vi "VI AK.vi"() -> (0 "error out":errorcluster)   [LabVIEW 2020, in "AK-Schnittstelle.lvlib"]
uses:
  AK-Schnittstelle.lvlib
  Aktionen AK.ctl
  Aktionen Gespeicherte Werte.ctl
  Allgemein/Zykluszeiterfassung Aktionen.ctl
  SysLog/SysLog Interface.ctl
  AK Seriell/AK Seriell.lvlib
  AK TCP/AK TCP.lvlib
  Allgemein/allgemeine Sub-VIs.lvlib
  SysLog/SysLog.lvlib
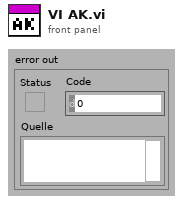
[diagram p1: front panel]
types:
  T1 = typedef "AK-Schnittstelle.lvlib/Aktionen AK.ctl" = enum16{"lesen", "initialisieren", "beenden", "AK Komm"}
  T2 = typedef "allgemeine Sub-VIs.lvlib/Zykluszeiterfassung Aktionen.ctl" = enum16{"lesen", "init", "Messdaten1", "ToolWeb", "AK FT-IR", "AK Extern", "AK Amium"}
  T3 = typedef "AK-Schnittstelle.lvlib/Aktionen Gespeicherte Werte.ctl" = enum16{"lesen", "laden", "speichern", "Seriell", "TCP", "Diverse", "AKTIV", "AK-Namen"}
  T4 = typedef "SysLog.lvlib/SysLog Interface.ctl" = cluster{"FehlermeldungsCode":i32, "ErfolgsmeldungsCode":i32, "ParameterListenString":string, "Anzeige":bool, "SysLogIcon":enum16{"OK", "Warnung", "Fehler"}, "intern":bool}
  T5 = typedef "AK-Schnittstelle.lvlib/AK TCP.lvlib/TCP Parameter.ctl" = cluster{"Port":u16, "Timeout":u16}
  T6 = typedef "AK-Schnittstelle.lvlib/AK Seriell.lvlib/Serielle Parameter.ctl" = cluster{"VISA resource name":refnum<visa-resource-name>, "baud rate":u32, "data bits":u16, "parity":u16, "stop bits":u16, "flow control":u16}
  T7 = cluster{"VISA resource name":bool, "baud rate":bool, "data bits":bool, "parity":bool, "stop bits":bool, "flow control":bool}
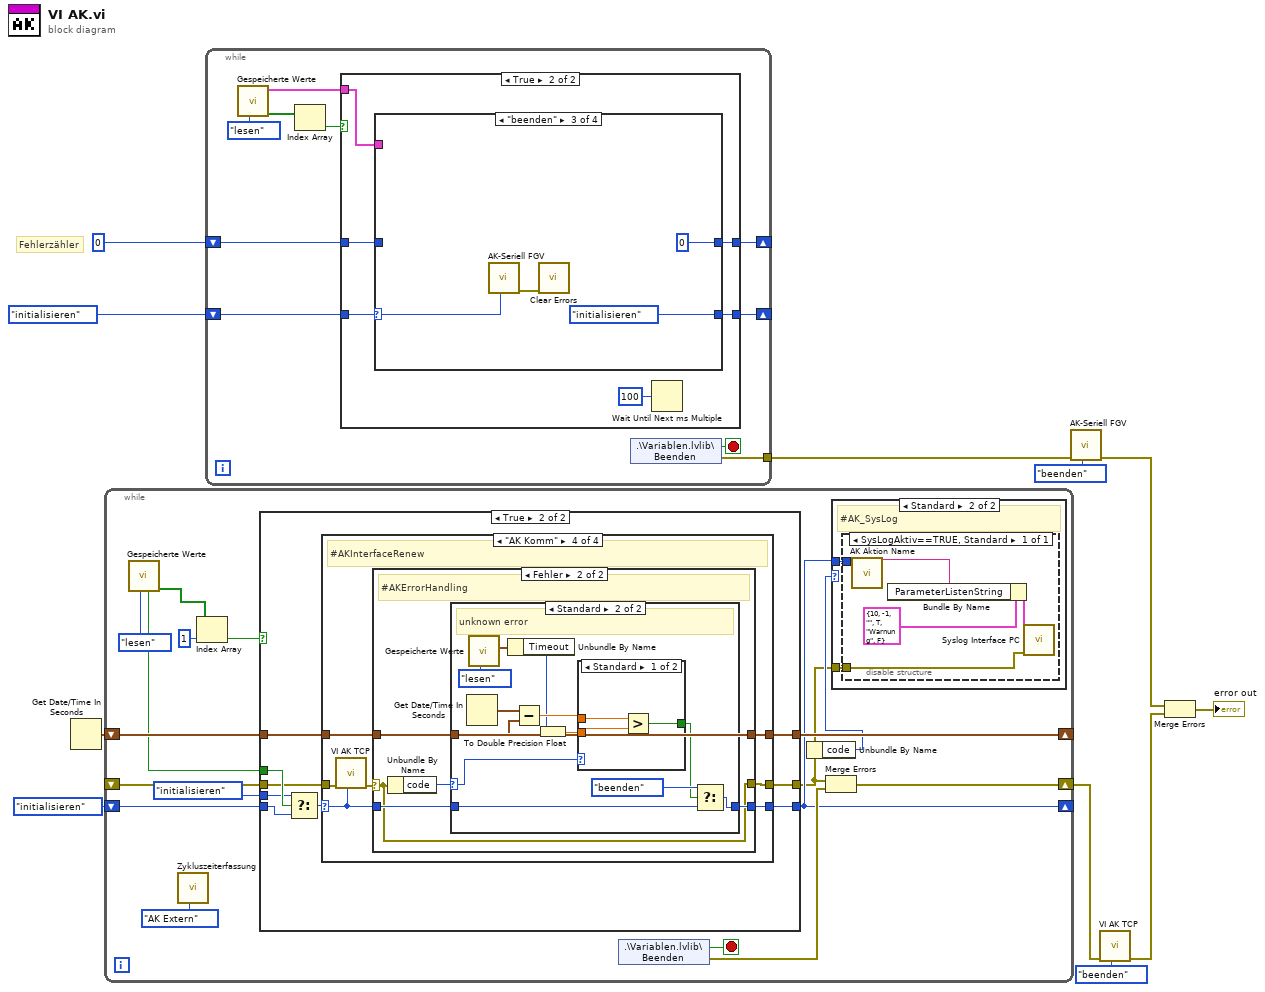
[diagram p0: block diagram]
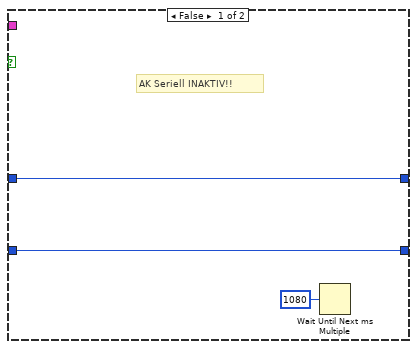
[diagram p2: hidden frame]
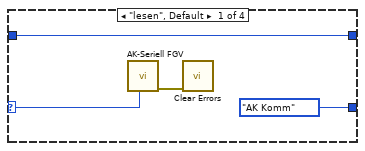
[diagram p3: hidden frame]
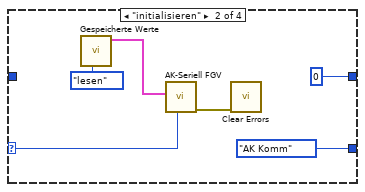
[diagram p4: hidden frame]
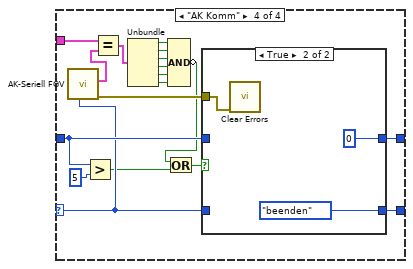
[diagram p5: hidden frame]
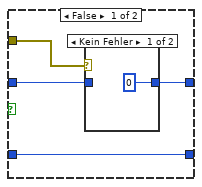
[diagram p6: hidden frame]
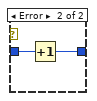
[diagram p7: hidden frame]
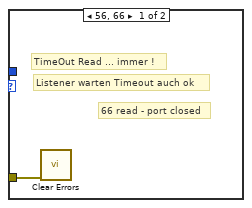
[diagram p8: hidden frame]
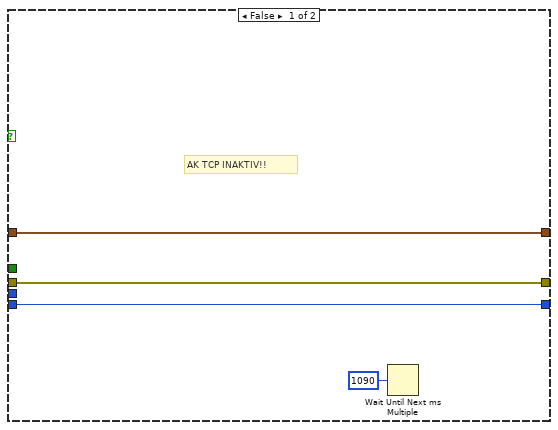
[diagram p9: hidden frame]
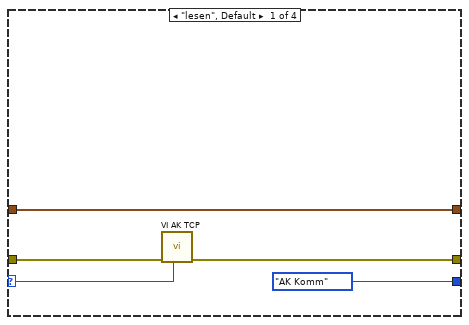
[diagram p10: hidden frame]
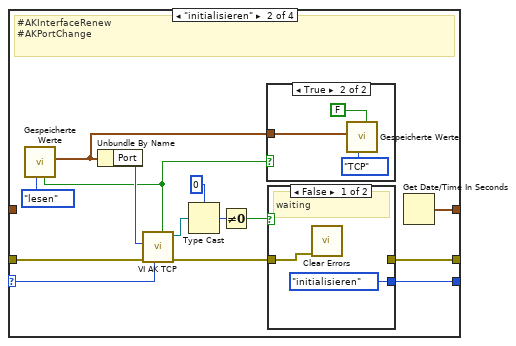
[diagram p11: hidden frame]
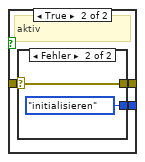
[diagram p12: hidden frame]
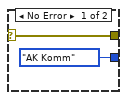
[diagram p13: hidden frame]
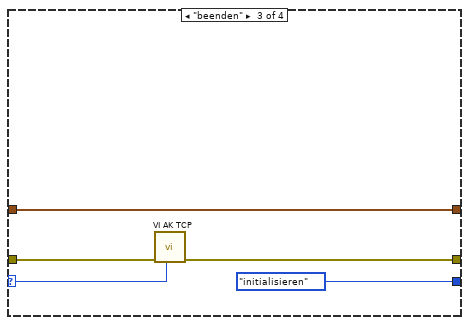
[diagram p15: hidden frame]
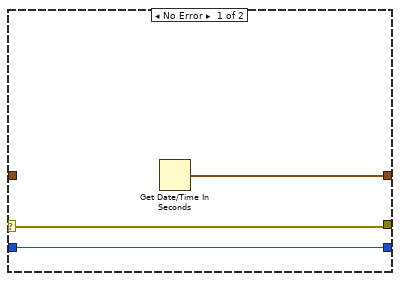
[diagram p16: hidden frame]
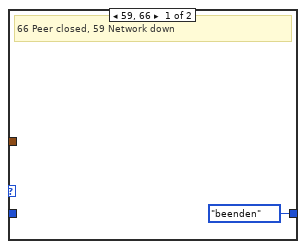
[diagram p17: hidden frame]
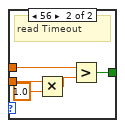
[diagram p18: hidden frame]
diagram:
  # "Fehlerzähler"
  n1 = Get Date/Time In Seconds() -> (seconds since 1Jan1904=w2:timestamp)
  n2 = while {
    shift-right: [w14] -> _
    shift-left: Aktionen_AK."initialisieren" ("Aktionen") -> [w28]
    shift-right: [w27] -> _
    shift-left: w2 -> [w26]
    shift-right: [w16] -> w1
    shift-left: _ -> [w15]
    stop <- w21 stop-if-true
    n3 = call "Gespeicherte Werte.vi"("Aktionen"=Aktionen_Gespeicherte_Werte."lesen") -> ("AKTIV?"=w24:bool[], "Port changed out"=w19:bool)  [unwired: 6 in, 3 out]
    n4 = call "Zykluszeiterfassung.vi"("Aktionen"=Zykluszeiterfassung_Aktionen."AK Extern") -> ()  [unwired: 10 in, 1 out]
    n5 = Index Array(array=w24, index=1 ("Index")) -> (element=w22:bool)
    n6 = case shown="True" w22 {
      tunnel: w28 -> [w39 w45]
      tunnel: [w39 w49] -> w14
      tunnel: [w40 w48] -> w27
      tunnel: w26 -> [w40 w47]
      tunnel: w19 -> [_ w46]
      tunnel: Aktionen_AK."initialisieren" ("Aktionen") -> [_ w44]
      tunnel: [w37 w42] -> w12
      tunnel: w15 -> [w37 w41]
      frame False {
        # "AK TCP INAKTIV!!"
        n7 = Wait Until Next ms Multiple(millisecond multiple=u32 1090 ("Vielfache von ms")) -> ()  [unwired: 1 out]
      }
      frame True {
        n8 = Select(t=w44, s=w46, f=w45) -> (s? t:f=w43:T1)
        n9 = case shown="\"AK Komm\"" w43 {
          selector: w43 -> [w52 w67 w84 w89]
          tunnel: [Aktionen_AK."AK Komm" ("Aktionen") w65 Aktionen_AK."initialisieren" ("Aktionen") w88] -> w49
          tunnel: [w53 w63 w83 w92] -> w48
          tunnel: w47 -> [w53 _ w83 w91]
          tunnel: [w50 w58 w81 w86] -> w42
          tunnel: w41 -> [w51 w57 w82 w87]
          frame "lesen", Default {
            n10 = call "VI AK TCP.vi"("Aktionen"=w52, "error in"=w51) -> ("error out"=w50:errorcluster)  [unwired: 8 in, 1 out]
          }
          frame "initialisieren" {
            # "#AKInterfaceRenew\n#AKPortChange"
            n11 = call "Gespeicherte Werte.vi"("Aktionen"=Aktionen_Gespeicherte_Werte."lesen") -> ("TCP Parameter"=w59:T5, "Port changed out"=w55:bool)  [unwired: 6 in, 3 out]
            n12 = Unbundle By Name(w59) -> ("Port"=w64:u16)
            n13 = call "VI AK TCP.vi"("Port changed in"=w55, "Aktionen"=w67, "error in"=w57, "Port"=w64) -> ("error out"=w66:errorcluster, "connection ID"=w56:refnum<k5>)  [unwired: 6 in]
            n14 = Type Cast(type=u32 0, x=w56) -> (*(type *) &x=w61:u32)
            n15 = Not Equal To 0?(x=w61) -> (x != 0?=w60:bool)
            n16 = case shown="True" w55 {
              tunnel: w59 -> [_ w78]
              frame False {
              }
              frame True {
                n17 = call "Gespeicherte Werte.vi"("Port changed in"=FALSE, "Aktionen"=Aktionen_Gespeicherte_Werte."TCP", "TCP Parameter"=w78) -> ()  [unwired: 4 in, 5 out]
              }
            }
            n18 = case shown="False" w60 {
              tunnel: w66 -> [w70 w73]
              tunnel: [Aktionen_AK."initialisieren" ("Aktionen") w72] -> w65
              tunnel: [_ w71] -> w58
              frame False {
                # "waiting"
                n19 = call <vilib>:"Clear Errors.vi"("error in (no error)"=w70) -> ()  [unwired: 5 in, 2 out]
              }
              frame True {
                # "aktiv"
                n20 = case shown="Fehler" w73 {
                  selector: w73 -> [w74 w76]
                  tunnel: [Aktionen_AK."AK Komm" ("Aktionen") Aktionen_AK."initialisieren" ("Aktionen")] -> w72
                  tunnel: [w74 w76] -> w71
                  frame No Error {
                  }
                  frame Error {
                  }
                }
              }
            }
            n21 = Get Date/Time In Seconds() -> (seconds since 1Jan1904=w63:timestamp)
          }
          frame "beenden" {
            n22 = call "VI AK TCP.vi"("Aktionen"=w84, "error in"=w82) -> ("error out"=w81:errorcluster)  [unwired: 8 in, 1 out]
          }
          frame "AK Komm" {
            # "#AKInterfaceRenew"
            n23 = call "VI AK TCP.vi"("Aktionen"=w89, "error in"=w87) -> ("error out"=w90:errorcluster)  [unwired: 8 in, 1 out]
            n24 = case shown="Fehler" w90 {
              selector: w90 -> [w93 w96]
              tunnel: [w95 w100] -> w92
              tunnel: w91 -> [_ w100]
              tunnel: w89 -> [w94 w99]
              tunnel: [w94 w98] -> w88
              tunnel: [w93 w96] -> w86
              frame No Error {
                n25 = Get Date/Time In Seconds() -> (seconds since 1Jan1904=w95:timestamp)
              }
              frame Error {
                # "#AKErrorHandling"
                n26 = Unbundle By Name(w96) -> ("code"=w97:i32)
                n27 = case shown="Standard" w97 {
                  selector: w97 -> [_ w105]
                  tunnel: w100 -> [_ w112]
                  tunnel: w99 -> [_ w109]
                  tunnel: [Aktionen_AK."beenden" ("Aktionen") w108] -> w98
                  frame 59, 66 {
                    # "66 Peer closed, 59 Network down"
                  }
                  frame Default {
                    # "unknown error"
                    n28 = Get Date/Time In Seconds() -> (seconds since 1Jan1904=w113:timestamp)
                    n29 = call "Gespeicherte Werte.vi"("Aktionen"=Aktionen_Gespeicherte_Werte."lesen") -> ("TCP Parameter"=w111:T5)  [unwired: 6 in, 4 out]
                    n30 = Unbundle By Name(w111) -> ("Timeout"=w103:u16)
                    n31 = Subtract(x=w113, y=w112) -> (x-y=w104:dbl)
                    n32 = To Double Precision Float(number=w103) -> (double precision float=w102:dbl)
                    n33 = case shown="Standard" w105 {
                      tunnel: w104 -> [w115 w121]
                      tunnel: w102 -> [w116 w120]
                      tunnel: [w114 w117] -> w106
                      frame Default {
                        n34 = Greater?(x=w115, y=w116) -> (0:w114:bool)
                      }
                      frame 56 {
                        # "read Timeout"
                        n35 = Multiply(x=w120, y=1.0) -> (x*y=w119:dbl)
                        n36 = Greater?(x=w121, y=w119) -> (0:w117:bool)
                      }
                    }
                    n37 = Select(t=Aktionen_AK."beenden" ("Aktionen"), s=w106, f=w109) -> (s? t:f=w108:T1)
                  }
                }
              }
            }
          }
        }
      }
    }
    n38 = shared-variable ".\\Variablen.lvlib\\Beenden"() -> (w21:bool, error out=w17:errorcluster)  [unwired: 1 in]
    n39 = Unbundle By Name(w12) -> ("code"=w13:i32)
    n40 = Merge Errors(w12, w17) -> (w16:errorcluster)
    n41 = case shown="Standard" w13 {
      tunnel: w14 -> [_ w31]
      tunnel: w12 -> [w29 w30]
      frame 56, 66 {
        # "66 read - port closed"
        # "Listener warten Timeout auch ok"
        # "TimeOut Read ... immer !"
        n42 = call <vilib>:"Clear Errors.vi"("error in (no error)"=w29) -> ()  [unwired: 5 in, 2 out]
      }
      frame Default {
        # "#AK_SysLog"
        n43 = disable-structure shown="SysLogAktiv==TRUE, Standard" {
          disable-tunnel: w31 -> [w36]
          disable-tunnel: w30 -> [w32]
          frame condition #0 (active) {
            n44 = call "AK Aktion Name.vi"("Aktionen"=w36) -> ("Aktions Name"=w33:string)  [unwired: 10 in]
            n45 = Bundle By Name(cluster=T4 {"FehlermeldungsCode"=10, "ErfolgsmeldungsCode"=-1, "ParameterListenString"="", "Anzeige"=TRUE, "SysLogIcon"=enum."Warnung", "intern"=FALSE} ("Cluster (in)"), "ParameterListenString"=w33) -> (w34:T4)
            n46 = call "Syslog Interface PC.vi"("Fehler (in)"=w32, "Cluster (in)"=w34) -> ()  [unwired: 9 in, 1 out]
          }
        }
      }
    }
  }
  n47 = while {
    shift-right: [w130] -> _
    shift-left: Aktionen_AK."initialisieren" ("Aktionen") -> [w131]
    shift-right: [w129] -> _
    shift-left: u8 0 -> [w128]
    tunnel: [w127] -> w3
    stop <- w123 stop-if-true
    n48 = call "Gespeicherte Werte.vi"("Aktionen"=Aktionen_Gespeicherte_Werte."lesen") -> ("AKTIV?"=w125:bool[], "Serielle Parameter"=w122:T6)  [unwired: 6 in, 3 out]
    n49 = Index Array(array=w125) -> (element=w124:bool)  [unwired: 1 in]
    n50 = case shown="True" w124 {
      tunnel: w131 -> [w132 w140]
      tunnel: [w132 w139] -> w130
      tunnel: [w134 w138] -> w129
      tunnel: w128 -> [w134 w137]
      tunnel: w122 -> [_ w135]
      frame False {
        # "AK Seriell INAKTIV!!"
        n51 = Wait Until Next ms Multiple(millisecond multiple=u32 1080 ("Vielfache von ms")) -> ()  [unwired: 1 out]
      }
      frame True {
        n52 = case shown="\"beenden\"" w140 {
          selector: w140 -> [w144 w150 w154 w168]
          tunnel: [Aktionen_AK."AK Komm" ("Aktionen") Aktionen_AK."AK Komm" ("Aktionen") Aktionen_AK."initialisieren" ("Aktionen") w169] -> w139
          tunnel: [w142 u8 0 u8 0 w172] -> w138
          tunnel: w137 -> [w142 _ _ w171]
          tunnel: w135 -> [_ _ _ w159]
          frame "lesen", Default {
            n53 = call "AK-Seriell FGV.vi"("Aktionen"=w144) -> ("error out"=w141:errorcluster)  [unwired: 9 in, 1 out]
            n54 = call <vilib>:"Clear Errors.vi"("error in (no error)"=w141) -> ()  [unwired: 5 in, 2 out]
          }
          frame "initialisieren" {
            n55 = call "Gespeicherte Werte.vi"("Aktionen"=Aktionen_Gespeicherte_Werte."lesen") -> ("Serielle Parameter"=w146:T6)  [unwired: 6 in, 4 out]
            n56 = call "AK-Seriell FGV.vi"("Aktionen"=w150, "Serielle Parameter"=w146) -> ("error out"=w145:errorcluster)  [unwired: 8 in, 1 out]
            n57 = call <vilib>:"Clear Errors.vi"("error in (no error)"=w145) -> ()  [unwired: 5 in, 2 out]
          }
          frame "beenden" {
            n58 = call "AK-Seriell FGV.vi"("Aktionen"=w154) -> ("error out"=w151:errorcluster)  [unwired: 9 in, 1 out]
            n59 = call <vilib>:"Clear Errors.vi"("error in (no error)"=w151) -> ()  [unwired: 5 in, 2 out]
          }
          frame "AK Komm" {
            n60 = call "AK-Seriell FGV.vi"("Aktionen"=w168) -> ("error out"=w167:errorcluster, "Serielle Parameter 2"=w158:T6)  [unwired: 9 in]
            n61 = Greater?(x=w171, y=u8 5) -> (0:w155:bool)
            n62 = Equal?(x=w159, y=w158) -> (x = y?=w166:T7)
            n63 = Unbundle(w166) -> ("VISA resource name"=w165:bool, "baud rate"=w164:bool, "data bits"=w163:bool, "parity"=w162:bool, "stop bits"=w161:bool, "flow control"=w160:bool)
            n64 = Compound Arithmetic op=AND ("Mehrfacharithmetik")(w165, w164, w163, w162, w161, w160) -> (invert w156:bool)
            n65 = Or(x=w156, y=w155) -> (x .or. y?=w157:bool)
            n66 = case shown="True" w157 {
              tunnel: [w176 u8 0] -> w172
              tunnel: w171 -> [w175 _]
              tunnel: w168 -> [w174 _]
              tunnel: [w174 Aktionen_AK."beenden" ("Aktionen")] -> w169
              tunnel: w167 -> [w173 w180]
              frame False {
                n67 = case shown="Kein Fehler" w173 {
                  tunnel: [u8 0 w179] -> w176
                  tunnel: w175 -> [_ w178]
                  frame No Error {
                  }
                  frame Error {
                    n68 = Increment(x=w178) -> (x+1=w179:u8)
                  }
                }
              }
              frame True {
                n69 = call <vilib>:"Clear Errors.vi"("error in (no error)"=w180) -> ()  [unwired: 5 in, 2 out]
              }
            }
          }
        }
        n70 = Wait Until Next ms Multiple(millisecond multiple=u32 100 ("Vielfache von ms")) -> ()  [unwired: 1 out]
      }
    }
    n71 = shared-variable ".\\Variablen.lvlib\\Beenden"() -> (w123:bool, error out=w127:errorcluster)  [unwired: 1 in]
  }
  n72 = call "AK-Seriell FGV.vi"("Aktionen"=Aktionen_AK."beenden", "error in"=w3) -> ("error out"=w11:errorcluster)  [unwired: 8 in, 1 out]
  n73 = call "VI AK TCP.vi"("Aktionen"=Aktionen_AK."beenden", "error in"=w1) -> ("error out"=w9:errorcluster)  [unwired: 8 in, 1 out]
  n74 = Merge Errors(w11, w9) -> (→"error out":errorcluster)
